vi "Upsert Attribute.vi"(0 "Attributes in":refnum<class "Attributes.lvclass">, 5 "Object ID":i32=-1, 7 "Key":string, 9 "Value":variant, 11 "error in (no error)":errorcluster) -> (4 "Attributes out":refnum<class "Attributes.lvclass">, 15 "error out":errorcluster)   [LabVIEW 2019, in "HierDAL Library.lvlib" / "Database.lvlib" / "Repositories.lvlib" / "Attributes.lvclass"]
uses:
  Attributes.lvclass
  Attributes.lvclass/Attributes.ctl
  Database Manager Class/Database Manager.lvclass
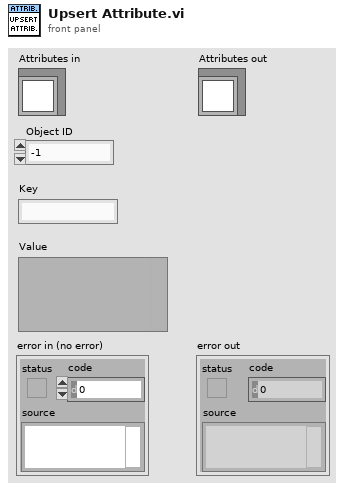
[diagram p1: front panel]
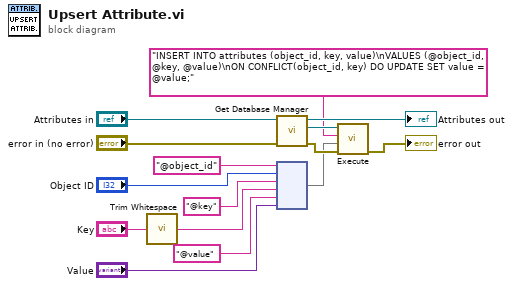
[diagram p0: block diagram]
diagram:
  n1 = call <vilib>:"Trim Whitespace.vi"("string"="Key") -> ("trimmed string"=w2:string)  [unwired: 1 in]
  n2 = call "Get Database Manager.vi"("error in (no error)"="error in (no error)", "Attributes in"="Attributes in") -> ("error out"=w8:errorcluster, "Database Manager"=w7:refnum<class "Database Manager.lvclass">, "Attributes out"=→"Attributes out":refnum<class "Attributes.lvclass">)  [unwired: 7 in]
  n3 = node("@object_id" ("key"), "Object ID", "@key" ("key"), w2, "@value" ("key"), "Value") -> (w5:map{string, variant})
  n4 = call-dynamic "Execute.vi"("error in (no error)"=w8, "Parameters"=w5, "Query"="INSERT INTO attributes (object_id, key, value)\nVALUES (@object_id, @key, @value)\nON CONFLICT(object_id, key) DO UPDATE SET value = @value;", "Database Manager in"=w7) -> ("error out"=→"error out":errorcluster)  [unwired: 5 in, 2 out]
